vi "Verify Spin time.vi"(0 "GEA2 Reference In":refnum<k24>, 5 "ECT Data In":T1, 11 "Error In":errorcluster) -> (3 "Expected SSD":string, 4 "GEA2 Reference Out":refnum<k24>, 6 "Actual ECT After Spin (sec)":u16, 8 "Expected ECT After Spin (sec)":u16, 10 "ECT After Spin Pass/Fail":bool, 14 "Report Text":string, 15 "Error Out":errorcluster)   [LabVIEW 2016, in "Centauro.lvlib"]
doc: "This vi can be used to read ERD every 1 sec for user selected repeat counts."
uses:
  Projects/Centauro.lvlib
  Common/LabVIEW GEA2 Toolkit/LabVIEW_GEA2_Toolkit.lvlibp/type defs/ERD Read Data In.ctl
  Common/LabVIEW GEA2 Toolkit/LabVIEW_GEA2_Toolkit.lvlibp
  Common/LabVIEW GEA2 Toolkit/LabVIEW_GEA2_Toolkit.lvlibp/type defs/Source_Destination.ctl
  Common/LabVIEW GEA2 Toolkit/LabVIEW_GEA2_Toolkit.lvlibp/type defs/Data Type.ctl
  Q:/Common/DLLs/GEA3/GeaCommunication.dll
  Common/DLLs/GEA3/GeaCommunication.dll
  Controls/ECT.ctl
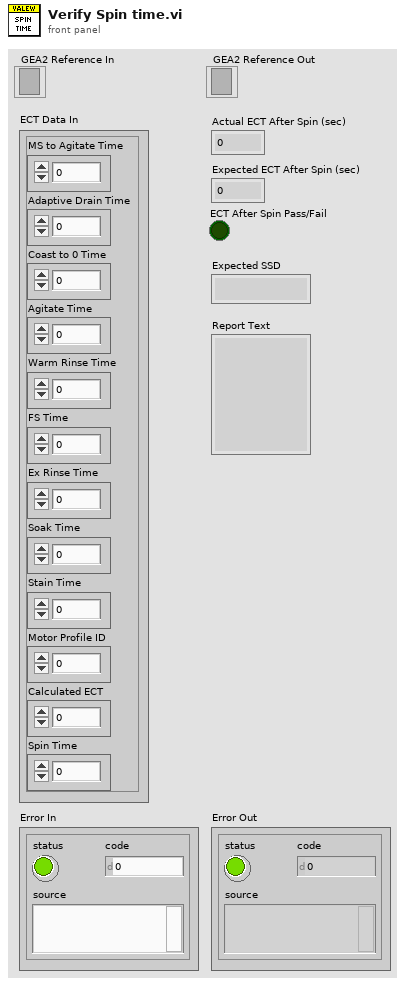
[diagram p1: front panel]
types:
  T1 = typedef "Centauro.lvlib/ECT.ctl" = cluster{"MS to Agitate Time":u16, "Adaptive Drain Time":u16, "Coast to 0 Time":u16, "Agitate Time":u16, "Warm Rinse Time":u16, "FS Time":u16, "Ex Rinse Time":u16, "Soak Time":u16, "Stain Time":u16, "Motor Profile ID":u16, "Calculated ECT":u16, "Spin Time":u16}
  T2 = typedef "LabVIEW_GEA2_Toolkit.lvlibp/Source_Destination.ctl" = cluster{"Source":u8, "Destination":u8}
  T3 = enum16{"EQ (==)", "NE (!=)", "GT (>)", "LT (<)", "GE (>=)", "LE (<=)", "GTLT(> <)", "GELE (>= <=)", "GELT (>= <)", "GTLE (> <=)", "LTGT (< >)", "LEGE (<= >=)", "LEGT (<= >)", "LTGE (< >=)", "No Comparison"}
  T4 = typedef "LabVIEW_GEA2_Toolkit.lvlibp/ERD Read Data In.ctl" = cluster{"ERD Number":u16, "Data Type":T5}
  T5 = typedef "LabVIEW_GEA2_Toolkit.lvlibp/Data Type.ctl" = enum16{"string", "boolean", "uint8_t", "uint16_t", "uint32_t", "uint64_t", "int8_t", "int16_t", "int32_t", "int64_t"}
  T6 = typedef "LabVIEW_GEA2_Toolkit.lvlibp/ERD Read Data Out.ctl" = cluster{"ERD Number":u16, "Data":string}
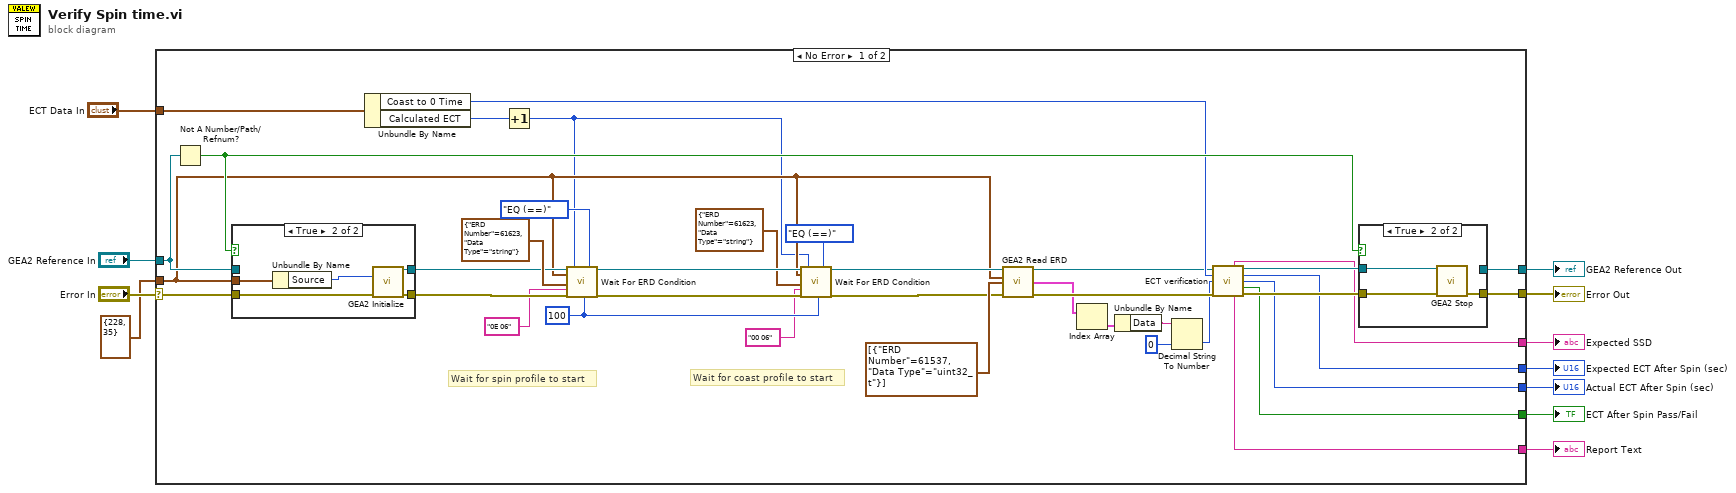
[diagram p0: block diagram]
diagram:
  n1 = case shown="No Error" "Error In" {
    selector: "Error In" -> [w48 w62]
    tunnel: T2 {"Source"=228, "Destination"=35} ("GEA Inputs") -> [w19 _]
    tunnel: "GEA2 Reference In" -> [w49 w63]
    tunnel: [w45 w63] -> w9
    tunnel: [w47 w62] -> w8
    tunnel: "ECT Data In" -> [w12 _]
    tunnel: [w42 _] -> w6
    tunnel: [w41 _] -> w5
    tunnel: [w40 _] -> w4
    tunnel: [w39 _] -> w3
    tunnel: [w38 _] -> w2
    frame No Error {
      w30 = u32 100 ("Loop Rate (ms)")
      # "Wait for coast profile to start"
      # "Wait for spin profile to start"
      n2 = Not A Number/Path/Refnum?(number/path/refnum=w49) -> (NaN/Path/Refnum?=w46:bool)
      n3 = case shown="True" w46 {
        tunnel: w48 -> [w56 w61]
        tunnel: [w56 w60] -> w20
        tunnel: [w55 w59] -> w21
        tunnel: w19 -> [_ w57]
        tunnel: w49 -> [w55 _]
        frame False {
        }
        frame True {
          n4 = Unbundle By Name(w57) -> ("Source"=w58:u8)
          n5 = call "GEA2 Initialize.vi"("Source Address"=w58, "error in"=w61) -> ("GEA2 Reference Out"=w59:refnum<k24>, "error out"=w60:errorcluster)  [unwired: 11 in, 1 out]
        }
      }
      n6 = Unbundle By Name(w12) -> ("Coast to 0 Time"=w37:u16, "Calculated ECT"=w17:u16)
      n7 = Increment(x=w17) -> (x+1=w16:u16)
      n8 = call "Wait For ERD Condition.vi"("GEA2 Reference In"=w21, "GEA Inputs"=w19, "ERD Read Data"=T4 {"ERD Number"=61623, "Data Type"=enum."string"}, "Expected Low"="0E 06" ("string"), "Error In"=w20, "Timeout (s)"=w16, "Loop Rate (ms)"=w30, "Comparison"=T3."EQ (==)") -> ("GEA2 Reference Out"=w33:refnum<k24>, "Error Out"=w32:errorcluster)  [unwired: 7 in, 3 out]
      n9 = call "Wait For ERD Condition.vi"("GEA2 Reference In"=w33, "GEA Inputs"=w19, "ERD Read Data"=T4 {"ERD Number"=61623, "Data Type"=enum."string"}, "Expected Low"="00 06" ("string"), "Error In"=w32, "Timeout (s)"=w16, "Loop Rate (ms)"=w30, "Comparison"=T3."EQ (==)") -> ("GEA2 Reference Out"=w31:refnum<k24>, "Error Out"=w18:errorcluster)  [unwired: 7 in, 3 out]
      n10 = call "GEA2 Read ERD.vi"("GEA2 Reference In"=w31, "GEA Inputs"=w19, "Read ERD List"=T4[] [{"ERD Number"=61537, "Data Type"=enum."uint32_t"}], "Error In"=w18) -> ("GEA2 Reference Out"=w27:refnum<k24>, "ERD Data Out"=w23:T6[], "Error Out"=w26:errorcluster)  [unwired: 8 in, 1 out]
      n11 = Index Array(array=w23) -> (element=w25:T6)  [unwired: 1 in]
      n12 = Unbundle By Name(w25) -> ("Data"=w24:string)
      n13 = Decimal String To Number(string=w24, default (0L)=u16 0 ("Actual ECT After Spin (sec)")) -> (number=w22:u16)  [unwired: 1 in, 1 out]
      n14 = call "ECT verification.vi"(".NET Refnum in"=w27, "Cal ECT (sec)"=w37, "Time remaining (sec)"=w22, "error in"=w26) -> ("Expected SSD"=w42:string, ".NET Refnum out"=w44:refnum<k24>, "Expected ECT (sec)"=w38:u16, "Actual ECT (sec)"=w40:u16, "ECT Pass/Fail"=w39:bool, "Report Text"=w41:string, "error out"=w43:errorcluster)  [unwired: 5 in]
      n15 = case shown="True" w46 {
        tunnel: [w51 w54] -> w47
        tunnel: w44 -> [w50 w53]
        tunnel: w43 -> [w51 w52]
        tunnel: [w50 _] -> w45
        frame False {
        }
        frame True {
          n16 = call "GEA2 Stop.vi"("GEA2 Reference In"=w53, "Error In"=w52) -> ("Error Out"=w54:errorcluster)  [unwired: 13 in]
        }
      }
    }
    frame Error {
    }
  }
  "GEA2 Reference Out" <- w9
  "Error Out" <- w8
  "Expected SSD" <- w6
  "Report Text" <- w5
  "Actual ECT After Spin (sec)" <- w4
  "ECT After Spin Pass/Fail" <- w3
  "Expected ECT After Spin (sec)" <- w2
